vi "includes.vi"   [LabVIEW 2013, in "Tag Bus Web Interface runtime.lvclass"]
uses:
  Tag Bus Web Interface runtime.lvclass
  configuration/Tag Bus Web Interface configuration.lvclass
  close.vi
  output.vi
  classify error.vi
  input.vi
  init.vi
  configuration/validate.vi
  configuration/to string.vi
  configuration/subtable.ctl
  configuration/from string.vi
  configuration/set channel.vi
  configuration/rename channel.vi
  configuration/get channels.vi
  configuration/delete channel from configuration.vi
  configuration/apply channel changes.vi
  configuration/add channel to configuration.vi
  configuration/data table to subtable.vi
  configuration/get supported types.vi
  configuration/Get Supported Targets.vi
  configuration/instance count allowed.vi
  configuration/execution class name.vi
  configuration/Write channels.vi
  configuration/Read channels.vi
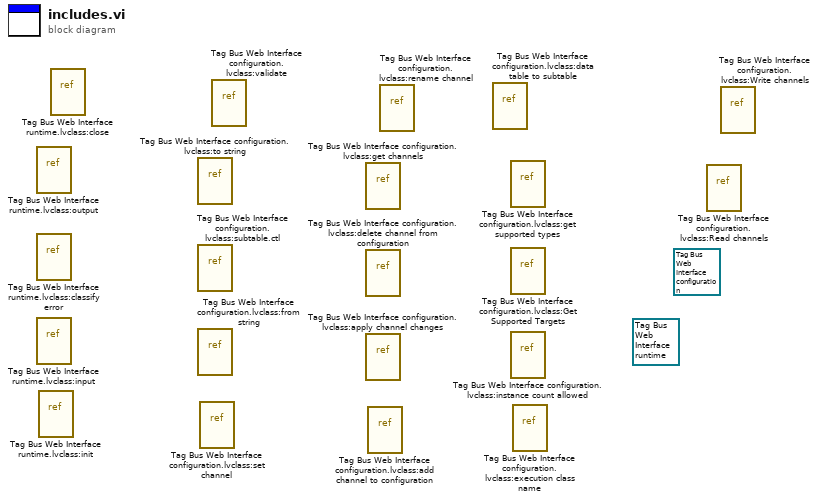
[diagram p0: block diagram]
diagram:
  (unwired) refnum<class "Tag Bus Web Interface configuration.lvclass"> refnum ("Tag Bus Web Interface configuration")
  (unwired) refnum<class "Tag Bus Web Interface runtime.lvclass"> refnum ("Tag Bus Web Interface runtime")
  n1 = vi-ref "Tag Bus Web Interface runtime.lvclass:output.vi"() -> ()  [unwired: 1 out]
  n2 = vi-ref "Tag Bus Web Interface runtime.lvclass:classify error.vi"() -> ()  [unwired: 1 out]
  n3 = vi-ref "Tag Bus Web Interface runtime.lvclass:input.vi"() -> ()  [unwired: 1 out]
  n4 = vi-ref "Tag Bus Web Interface runtime.lvclass:init.vi"() -> ()  [unwired: 1 out]
  n5 = vi-ref "Tag Bus Web Interface runtime.lvclass:close.vi"() -> ()  [unwired: 1 out]
  n6 = vi-ref "Tag Bus Web Interface configuration.lvclass:to string.vi"() -> ()  [unwired: 1 out]
  n7 = vi-ref "Tag Bus Web Interface configuration.lvclass:subtable.ctl"() -> ()  [unwired: 1 out]
  n8 = vi-ref "Tag Bus Web Interface configuration.lvclass:from string.vi"() -> ()  [unwired: 1 out]
  n9 = vi-ref "Tag Bus Web Interface configuration.lvclass:set channel.vi"() -> ()  [unwired: 1 out]
  n10 = vi-ref "Tag Bus Web Interface configuration.lvclass:validate.vi"() -> ()  [unwired: 1 out]
  n11 = vi-ref "Tag Bus Web Interface configuration.lvclass:get channels.vi"() -> ()  [unwired: 1 out]
  n12 = vi-ref "Tag Bus Web Interface configuration.lvclass:delete channel from configuration.vi"() -> ()  [unwired: 1 out]
  n13 = vi-ref "Tag Bus Web Interface configuration.lvclass:apply channel changes.vi"() -> ()  [unwired: 1 out]
  n14 = vi-ref "Tag Bus Web Interface configuration.lvclass:add channel to configuration.vi"() -> ()  [unwired: 1 out]
  n15 = vi-ref "Tag Bus Web Interface configuration.lvclass:rename channel.vi"() -> ()  [unwired: 1 out]
  n16 = vi-ref "Tag Bus Web Interface configuration.lvclass:data table to subtable.vi"() -> ()  [unwired: 1 out]
  n17 = vi-ref "Tag Bus Web Interface configuration.lvclass:get supported types.vi"() -> ()  [unwired: 1 out]
  n18 = vi-ref "Tag Bus Web Interface configuration.lvclass:Get Supported Targets.vi"() -> ()  [unwired: 1 out]
  n19 = vi-ref "Tag Bus Web Interface configuration.lvclass:instance count allowed.vi"() -> ()  [unwired: 1 out]
  n20 = vi-ref "Tag Bus Web Interface configuration.lvclass:execution class name.vi"() -> ()  [unwired: 1 out]
  n21 = vi-ref "Tag Bus Web Interface configuration.lvclass:Read channels.vi"() -> ()  [unwired: 1 out]
  n22 = vi-ref "Tag Bus Web Interface configuration.lvclass:Write channels.vi"() -> ()  [unwired: 1 out]
